vi "process kalman results.vi"(8 "reset graphs":bool, 9 "feedback lowpass f":dbl=30.0 format="%0.4f", 10 "graph lowpass f":dbl=30.0 format="%0.4f", 11 "kalman updates":T1[](array[typedef])) -> (1 "photon graphs":cluster{"t":dbl[], "x":dbl[]}[](array[cluster]), 2 "vel graphs":cluster{"t":dbl[], "v":dbl[]}[](array[cluster]), 3 "pos graphs":cluster{"t":dbl[], "x":dbl[]}[](array[cluster]), 4 "current velocity":dbl[](array[numeric]), 5 "current position":dbl[](array[numeric]))   [LabVIEW 2010]
uses:
  kalman_result_scaled.ctl
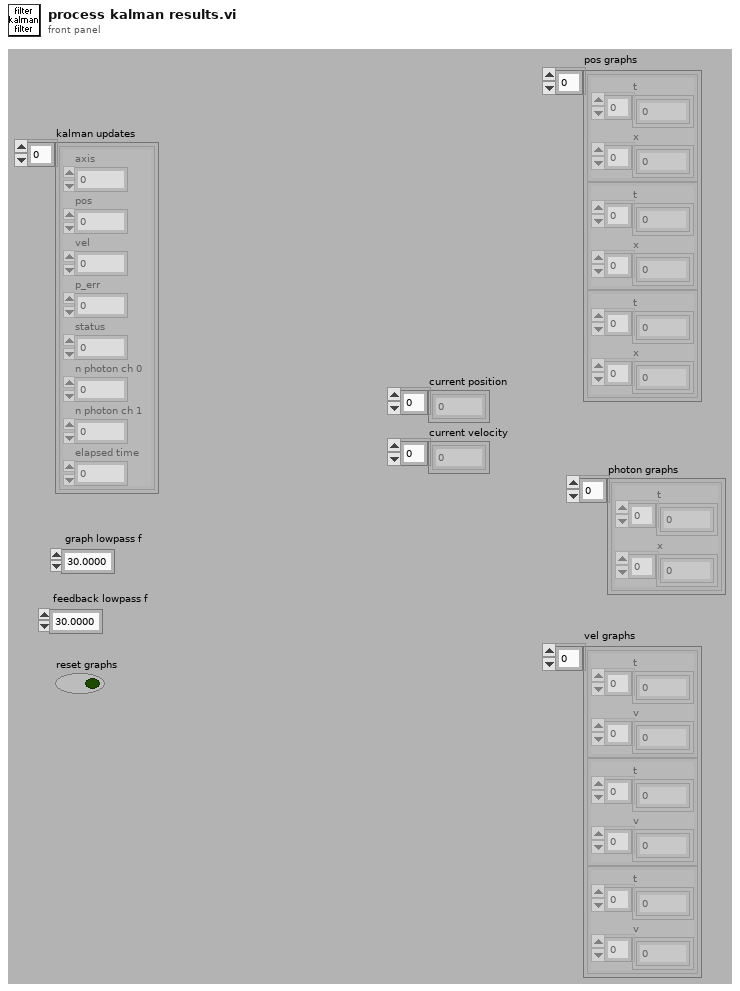
[diagram p1: front panel]
types:
  T1 = typedef "kalman_result_scaled.ctl" = cluster{"axis":u8, "pos":dbl, "vel":dbl, "p_err":dbl, "status":u32, "n photon ch 0":u32, "n photon ch 1":u32, "elapsed time":dbl}
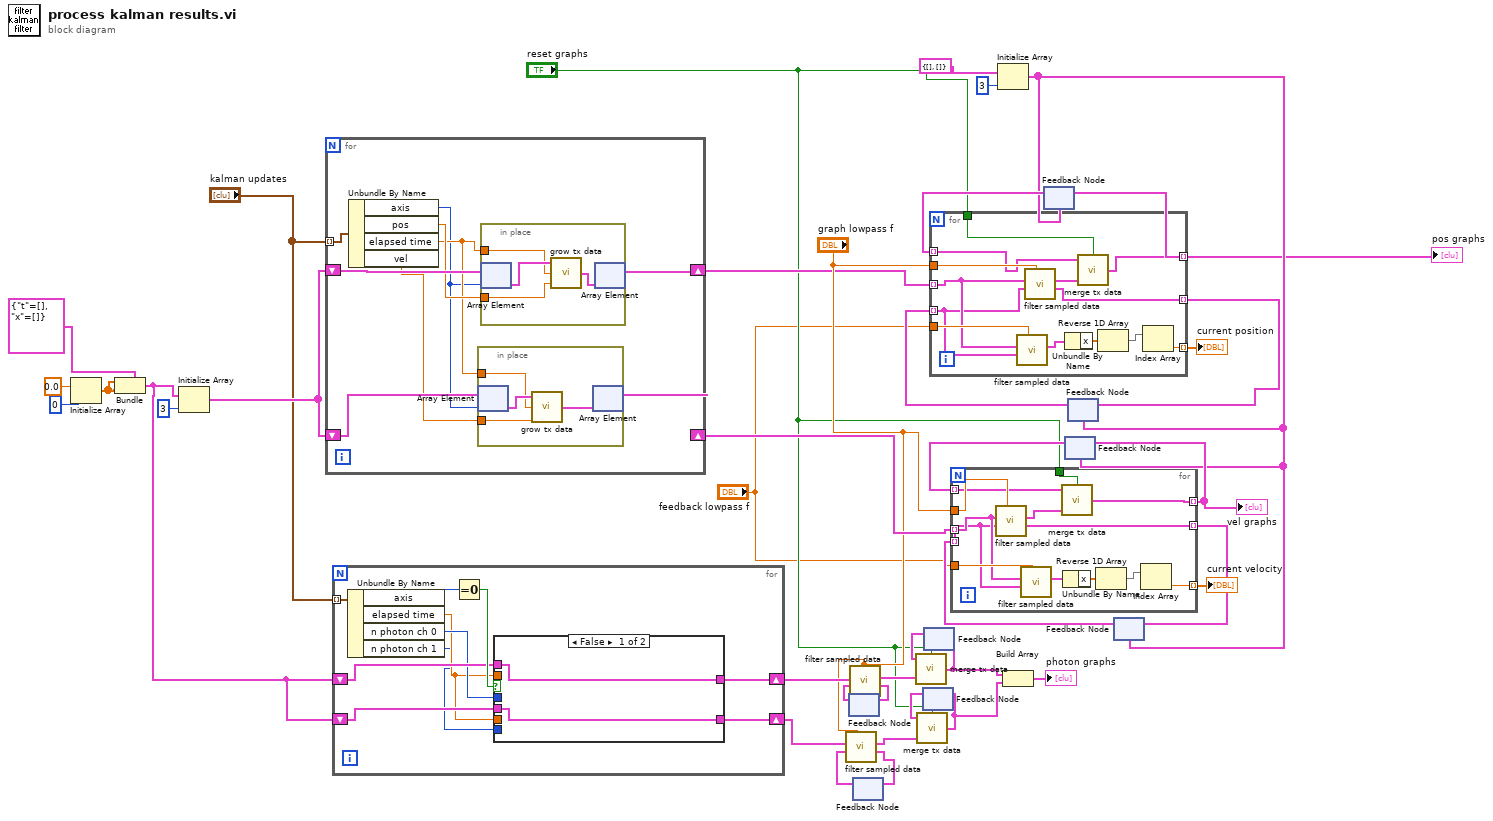
[diagram p0: block diagram]
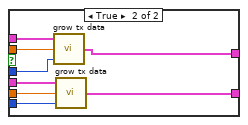
[diagram p2: hidden frame]
diagram:
  n1 = Initialize Array(0.0 ("element"), 0 ("dimension size")) -> (w29:dbl[])
  n2 = Bundle(cluster=cluster{"t":dbl[], "x":dbl[]} {"t"=[], "x"=[]} ("xt val"), "t"=w29, "x"=w29) -> (w22:cluster{"t":dbl[], "x":dbl[]})
  n3 = Initialize Array(w22, 3 ("dimension size")) -> (w38:cluster{"t":dbl[], "x":dbl[]}[])
  n4 = for {
    tunnel: "kalman updates" -> [w40] mode=indexing
    shift-right: [w46] -> w7
    shift-left: w38 -> [w48]
    shift-right: [w41] -> w35
    shift-left: w38 -> [w45]
    n5 = Unbundle By Name(w40) -> ("axis"=w42:u8, "pos"=w47:dbl, "elapsed time"=w44:dbl, "vel"=w43:dbl)
    n6 = in-place {
      in-place-border: w44 -> [w51]
      in-place-border: w43 -> [w50]
      n7 = in-place-array #1(w45, w42) -> (w52:cluster{"t":dbl[], "x":dbl[]})
      n8 = call "grow tx data.vi"("value"=w50, "time"=w51, "tx data in"=w52) -> ("tx data out"=w49:cluster{"t":dbl[], "x":dbl[]})
      n9 = in-place-array #1(w49) -> (w41:cluster{"t":dbl[], "x":dbl[]}[])  [unwired: 1 out]
    }
    n10 = in-place {
      in-place-border: w44 -> [w55]
      in-place-border: w47 -> [w54]
      n11 = in-place-array #2(w48, w42) -> (w56:cluster{"t":dbl[], "x":dbl[]})
      n12 = call "grow tx data.vi"("value"=w54, "time"=w55, "tx data in"=w56) -> ("tx data out"=w53:cluster{"t":dbl[], "x":dbl[]})
      n13 = in-place-array #2(w53) -> (w46:cluster{"t":dbl[], "x":dbl[]}[])  [unwired: 1 out]
    }
  }
  n14 = for {
    tunnel: "kalman updates" -> [w66] mode=indexing
    shift-right: [w62] -> w21
    shift-left: w22 -> [w63]
    shift-right: [w60] -> w18
    shift-left: w22 -> [w61]
    n15 = Unbundle By Name(w66) -> ("axis"=w65:u8, "elapsed time"=w58:dbl, "n photon ch 0"=w59:u32, "n photon ch 1"=w57:u32)
    n16 = Equal To 0?(x=w65) -> (x = 0?=w64:bool)
    n17 = case shown="False" w64 {
      tunnel: w63 -> [w68 w76]
      tunnel: [w68 w75] -> w62
      tunnel: w61 -> [w67 w74]
      tunnel: [w67 w73] -> w60
      tunnel: w58 -> [_ w72]
      tunnel: w59 -> [_ w71]
      tunnel: w58 -> [_ w70]
      tunnel: w57 -> [_ w69]
      frame False {
      }
      frame True {
        n18 = call "grow tx data.vi"("value"=w71, "time"=w72, "tx data in"=w76) -> ("tx data out"=w75:cluster{"t":dbl[], "x":dbl[]})
        n19 = call "grow tx data.vi"("value"=w69, "time"=w70, "tx data in"=w74) -> ("tx data out"=w73:cluster{"t":dbl[], "x":dbl[]})
      }
    }
  }
  n20 = feedback #3() -> (w19:cluster{"t":dbl[], "x":dbl[]})  [unwired: 1 in]
  n21 = call "filter sampled data.vi"("low cutoff freq: fl"="graph lowpass f", "last data set"=w19, "t x data"=w21) -> ("current data set"=w20:cluster{"t":dbl[], "x":dbl[]}, "t x data filetered"=w13:cluster{"t":dbl[], "x":dbl[]})  [unwired: 7 in]
  n22 = feedback-in #3(w20) -> ()
  n23 = feedback #4() -> (w16:cluster{"t":dbl[], "x":dbl[]})  [unwired: 1 in]
  n24 = call "filter sampled data.vi"("low cutoff freq: fl"="graph lowpass f", "last data set"=w16, "t x data"=w18) -> ("current data set"=w17:cluster{"t":dbl[], "x":dbl[]}, "t x data filetered"=w14:cluster{"t":dbl[], "x":dbl[]})  [unwired: 7 in]
  n25 = feedback-in #4(w17) -> ()
  n26 = feedback #5() -> (w11:cluster{"t":dbl[], "x":dbl[]})  [unwired: 1 in]
  n27 = call "merge tx data.vi"("do not merge"="reset graphs", "tx data new"=w14, "tx data in"=w11) -> ("tx data out"=w9:cluster{"t":dbl[], "x":dbl[]})  [unwired: 1 in]
  n28 = feedback-in #5(w9) -> ()
  n29 = feedback #6() -> (w12:cluster{"t":dbl[], "x":dbl[]})  [unwired: 1 in]
  n30 = call "merge tx data.vi"("do not merge"="reset graphs", "tx data new"=w13, "tx data in"=w12) -> ("tx data out"=w10:cluster{"t":dbl[], "x":dbl[]})  [unwired: 1 in]
  n31 = feedback-in #6(w10) -> ()
  n32 = Initialize Array(cluster{"t":dbl[], "x":dbl[]} {"t"=[], "x"=[]} ("xt val"), 3 ("dimension size")) -> (w23:cluster{"t":dbl[], "x":dbl[]}[])
  n33 = Build Array(w10, w9) -> (→"photon graphs":cluster{"t":dbl[], "x":dbl[]}[])
  n34 = feedback #7(w23) -> (w37:cluster{"t":dbl[], "x":dbl[]}[])
  n35 = feedback #8(w23) -> (w36:cluster{"t":dbl[], "x":dbl[]}[])
  n36 = feedback #9(w23) -> (w26:cluster{"t":dbl[], "x":dbl[]}[])
  n37 = for {
    tunnel: w7 -> [w82] mode=indexing
    tunnel: [w85] -> w6 mode=indexing
    tunnel: "graph lowpass f" -> [w89]
    tunnel: w37 -> [w87] mode=indexing
    tunnel: [w88] -> w27 mode=indexing
    tunnel: w26 -> [w81] mode=indexing
    tunnel: "reset graphs" -> [w84]
    tunnel: "feedback lowpass f" -> [w83]
    tunnel: [w77] -> w4 mode=indexing
    n38 = call "filter sampled data.vi"("low cutoff freq: fl"=w83, "last data set"=w81, "t x data"=w82) -> ("t x data filetered"=w80:cluster{"t":dbl[], "x":dbl[]})  [unwired: 7 in, 1 out]
    n39 = call "filter sampled data.vi"("low cutoff freq: fl"=w89, "last data set"=w81, "t x data"=w82) -> ("current data set"=w88:cluster{"t":dbl[], "x":dbl[]}, "t x data filetered"=w86:cluster{"t":dbl[], "x":dbl[]})  [unwired: 7 in]
    n40 = Unbundle By Name(w80) -> ("x"=w78:dbl[])
    n41 = call "merge tx data.vi"("do not merge"=w84, "tx data new"=w86, "tx data in"=w87) -> ("tx data out"=w85:cluster{"t":dbl[], "x":dbl[]})  [unwired: 1 in]
    n42 = Reverse 1D Array(array=w78) -> (reversed array=w79:dbl[])
    n43 = Index Array(array=w79) -> (element=w77:dbl)  [unwired: 1 in]
  }
  "pos graphs" <- w6
  "current position" <- w4
  n44 = feedback-in #7(w6) -> ()
  n45 = feedback-in #9(w27) -> ()
  n46 = feedback #10(w23) -> (w24:cluster{"t":dbl[], "x":dbl[]}[])
  n47 = for {
    tunnel: w35 -> [w95] mode=indexing
    tunnel: [w98] -> w32 mode=indexing
    tunnel: "graph lowpass f" -> [w102]
    tunnel: w36 -> [w99] mode=indexing
    tunnel: [w101] -> w25 mode=indexing
    tunnel: w24 -> [w94] mode=indexing
    tunnel: "reset graphs" -> [w97]
    tunnel: "feedback lowpass f" -> [w96]
    tunnel: [w90] -> w2 mode=indexing
    n48 = call "filter sampled data.vi"("low cutoff freq: fl"=w102, "last data set"=w94, "t x data"=w95) -> ("current data set"=w101:cluster{"t":dbl[], "x":dbl[]}, "t x data filetered"=w100:cluster{"t":dbl[], "x":dbl[]})  [unwired: 7 in]
    n49 = call "filter sampled data.vi"("low cutoff freq: fl"=w96, "last data set"=w94, "t x data"=w95) -> ("t x data filetered"=w91:cluster{"t":dbl[], "x":dbl[]})  [unwired: 7 in, 1 out]
    n50 = call "merge tx data.vi"("do not merge"=w97, "tx data new"=w100, "tx data in"=w99) -> ("tx data out"=w98:cluster{"t":dbl[], "x":dbl[]})  [unwired: 1 in]
    n51 = Unbundle By Name(w91) -> ("x"=w92:dbl[])
    n52 = Reverse 1D Array(array=w92) -> (reversed array=w93:dbl[])
    n53 = Index Array(array=w93) -> (element=w90:dbl)  [unwired: 1 in]
  }
  "vel graphs" <- w32
  "current velocity" <- w2
  n54 = feedback-in #8(w32) -> ()
  n55 = feedback-in #10(w25) -> ()
